vi "timer1.vi"(1 "Numeric 2":dbl=300.0) -> ()   [LabVIEW 2021]
panel:
  in  "Numeric":dbl
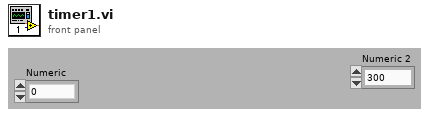
[diagram p1: front panel]
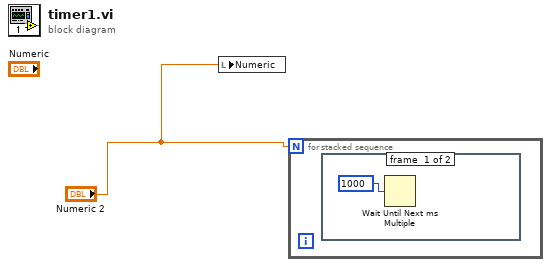
[diagram p0: block diagram]
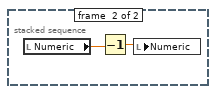
[diagram p2: hidden frame]
diagram:
  n1 = local write "Numeric"("Numeric 2") -> ()
  n2 = for {
    N: "Numeric 2" -> [_]
    n3 = stacked-sequence {
      frame #0 {
        n4 = Wait Until Next ms Multiple(millisecond multiple=u32 1000 ("millisecond timer value")) -> ()  [unwired: 1 out]
      }
      frame #1 {
        n5 = local read "Numeric"() -> (w4:dbl)
        n6 = Decrement(x=w4) -> (x-1=w3:dbl)
        n7 = local write "Numeric"(w3) -> ()
      }
    }
  }
